vi "controls_visible_status.vi"(10 "controls":refnum<vi>[](array[refnum]), 11 "status":bool) -> ()   [LabVIEW 2016, in "MotionControl.lvlib"]
uses:
  <userlib>/MotionControl/MotionControl.lvlib
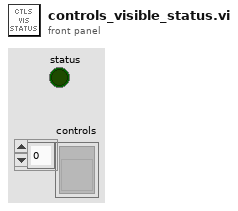
[diagram p1: front panel]
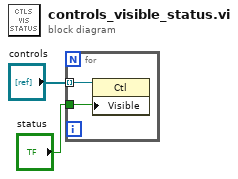
[diagram p0: block diagram]
diagram:
  n1 = for {
    tunnel: "status" -> [w3]
    tunnel: "controls" -> [w4] mode=indexing
    n2 = property class="Ctl"(reference=w4, "Visible"=w3) -> ()  [unwired: 1 in, 2 out]
  }
